vi "Report.vi"(1 "mesagge":string, 2 "client":string) -> ()   [LabVIEW 2010]
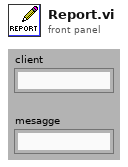
[diagram p1: front panel]
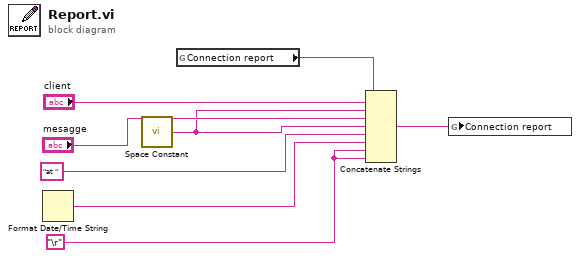
[diagram p0: block diagram]
diagram:
  w4 = "\r"
  n1 = Format Date/Time String() -> (date/time string=w5:string)  [unwired: 3 out]
  n2 = call <vilib>:"Space Constant.vi"() -> ("String"=w1:string)
  n3 = global read "ConnectionReport.vi" "Connection report"() -> (w3:string)
  n4 = Concatenate Strings(w3, "client", w1, "mesagge", w1, "at " ("string"), w5, w4, w4) -> (w8:string)
  n5 = global write "ConnectionReport.vi" "Connection report"(w8) -> ()
